vi "Check Status.vi"(8 "error in (no error)":errorcluster, 11 "Anritsu Optical Power Meter  in":refnum<class "Anritsu Optical Power Meter .lvclass">) -> (0 "error out":errorcluster, 1 "Status":string, 2 "Ready?":bool, 3 "Anritsu Optical Power Meter  out":refnum<class "Anritsu Optical Power Meter .lvclass">)   [LabVIEW 2017, in "Anritsu Optical Power Meter .lvclass"]
doc: "(Dynamic) Check if the instrument is powered on and update its member fields with the instrument's current status. Optionally return a text status message."
uses:
  Anritsu Optical Power Meter .lvclass
  Anritsu Power Meter/Public/Display control.ctl
  Anritsu Optical Power Meter .lvclass/Anritsu Optical Power Meter .ctl
  Utility Classes/Readable/Readable.lvclass
  <vilib>/regexp/Match Regular Expression.xnode
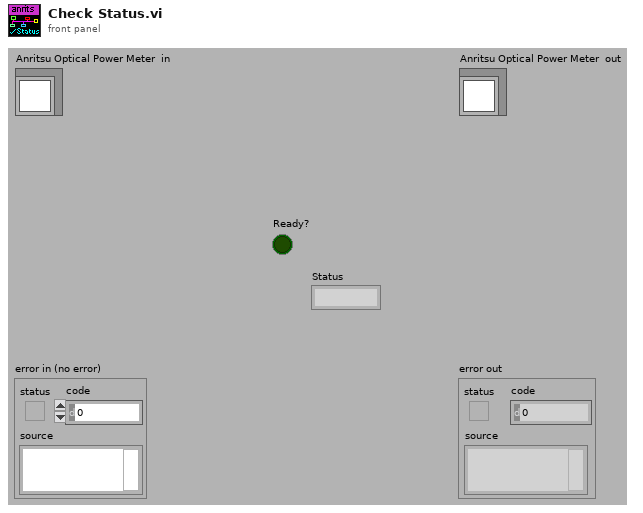
[diagram p1: front panel]
types:
  T1 = typedef "Display control.ctl" = enum16{"Watt", "dBm", "dB (REL)"}
  T2 = typedef "Range control watts and dBm.ctl" = enum16{"10 mW (+10 dBm)", "1 mW (0 dBm)", "100 uW (-10 dBm)", "10 uW (-20 dBm)", "1 uW (-30 dBm)", "100 nW (-40 dBm)", "10 nW (-50 dBm)", "1 nW (-60 dBm)", "100 pW (-70 dBm)", "10 pW (-80 dBm)"}
  T3 = typedef "Averaging control.ctl" = enum16{"On", "Off"}
  T4 = typedef "Auto Range control.ctl" = enum16{"Off", "On"}
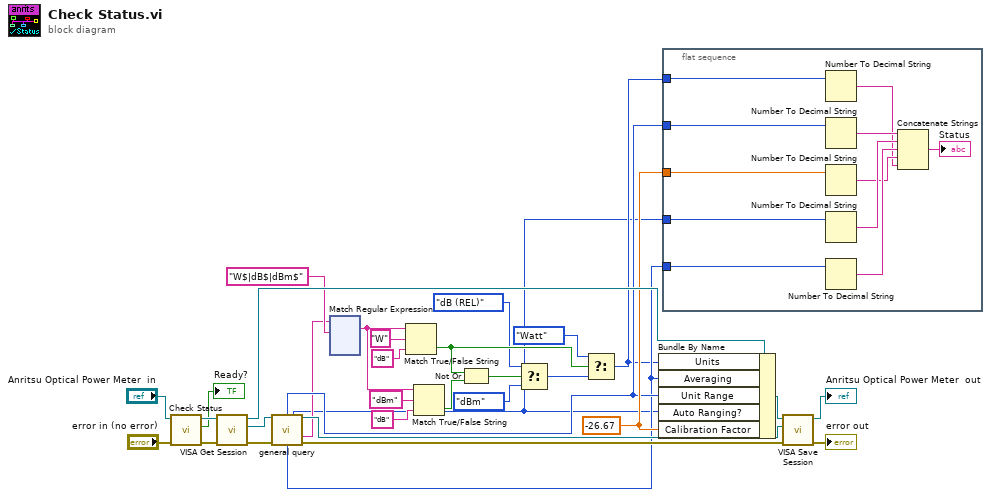
[diagram p0: block diagram]
diagram:
  w19 = -26.67 ("Calibration Factor")
  n1 = call-parent "Check Status.vi"("error in (no error)"="error in (no error)", "Instrument in"="Anritsu Optical Power Meter  in") -> ("error out"=w30:errorcluster, "Ready?"=→"Ready?":bool, "Instrument out"=w29:refnum<class "Anritsu Optical Power Meter .lvclass">)  [unwired: 6 in, 1 out]
  n2 = call-dynamic "VISA Get Session.vi"("error in (no error)"=w30, "Instrument.lvclass in"=w29) -> ("error out"=w26:errorcluster, "VISA Resource Name"=w27:refnum<visa-resource-name>, "Instrument.lvclass out"=w25:refnum<class "Anritsu Optical Power Meter .lvclass">)  [unwired: 7 out]
  n3 = call "general query.vi"("VISA resource name"=w27, "error in (no error)"=w26) -> ("Range W and dBm"=w18:T2, "VISA resource name out"=w23:refnum<visa-resource-name>, "Units"=w3:string, "Averaging"=w17:T3, "Auto Ranging?"=w1:T4, "error out"=w22:errorcluster)  [unwired: 5 in, 3 out]
  n4 = xnode "Match Regular Expression"("input string"=w3, "regular expression"="W$|dB$|dBm$") -> ("whole match"=w13:string)  [unwired: 4 in, 4 out]
  n5 = Match True/False String(2:"dB" ("false string"), 3:"W", 4:w13) -> (0:w9:bool)  [unwired: 1 out]
  n6 = Match True/False String(2:"dB" ("false string"), 3:"dBm" ("true string"), 4:w13) -> (0:w10:bool)  [unwired: 1 out]
  n7 = Not Or(1:w10, 2:w9) -> (0:w7:bool)
  n8 = Select(t=Display_control."dB (REL)" ("Display Units"), s=w7, f=Display_control."dBm" ("Display Units")) -> (s? t:f=w4:T1)
  n9 = Select(t=Display_control."Watt" ("Display Units"), s=w9, f=w4) -> (s? t:f=w2:T1)
  n10 = Bundle By Name(cluster=w25, "Units"=w2, "Averaging"=w17, "Unit Range"=w18, "Auto Ranging?"=w1, "Calibration Factor"=w19) -> (w24:refnum<class "Anritsu Optical Power Meter .lvclass">)
  n11 = flat-sequence {
    tunnel: w17 -> [w41]
    tunnel: w19 -> [w43]
    tunnel: w2 -> [w40]
    tunnel: w18 -> [w42]
    tunnel: w1 -> [w33]
    frame #0 {
      n12 = Number To Decimal String(number=w40) -> (decimal integer string=w35:string)  [unwired: 1 in]
      n13 = Number To Decimal String(number=w42) -> (decimal integer string=w39:string)  [unwired: 1 in]
      n14 = Number To Decimal String(number=w43) -> (decimal integer string=w36:string)  [unwired: 1 in]
      n15 = Number To Decimal String(number=w33) -> (decimal integer string=w38:string)  [unwired: 1 in]
      n16 = Number To Decimal String(number=w41) -> (decimal integer string=w37:string)  [unwired: 1 in]
      n17 = Concatenate Strings(w39, w38, w37, w36, w35) -> (→"Status":string)
    }
  }
  n18 = call-dynamic "VISA Save Session.vi"("error in (no error)"=w22, "VISA Resource Name"=w23, "Instrument.lvclass in"=w24) -> ("error out"=→"error out":errorcluster, "Instrument.lvclass out"=→"Anritsu Optical Power Meter  out":refnum<class "Anritsu Optical Power Meter .lvclass">)  [unwired: 7 out]
